vi "Create Arrow.vi"(6 "Quiver Size":sgl, 7 "Scale":cluster{"X":sgl, "Y":sgl, "Z":sgl}, 8 "error in (no error)":errorcluster, 9 "Color Array":cluster{"R":sgl, "G":sgl, "B":sgl, "A":sgl}[](array[cluster]), 10 "Normal Vertex":cluster{"X":sgl, "Y":sgl, "Z":sgl}[](array[cluster]), 11 "Quiver Object In":refnum<vi>) -> (0 "error out":errorcluster, 3 "Quiver Object Out":refnum<vi>)   [LabVIEW 2017, in "3D Quiver.lvclass"]
uses:
  <vilib>/Math Plots/3D Math Plots/3D Quiver/3D Quiver/3D Quiver.lvclass
  <vilib>/picture/3D Picture Control/Object/Create Object (name).vi
  <vilib>/picture/3D Picture Control/NI_3D Picture Control.lvlib
  <vilib>/Math Plots/3D Math Plots/3D Plot/3D Plot/3D Plot.lvclass
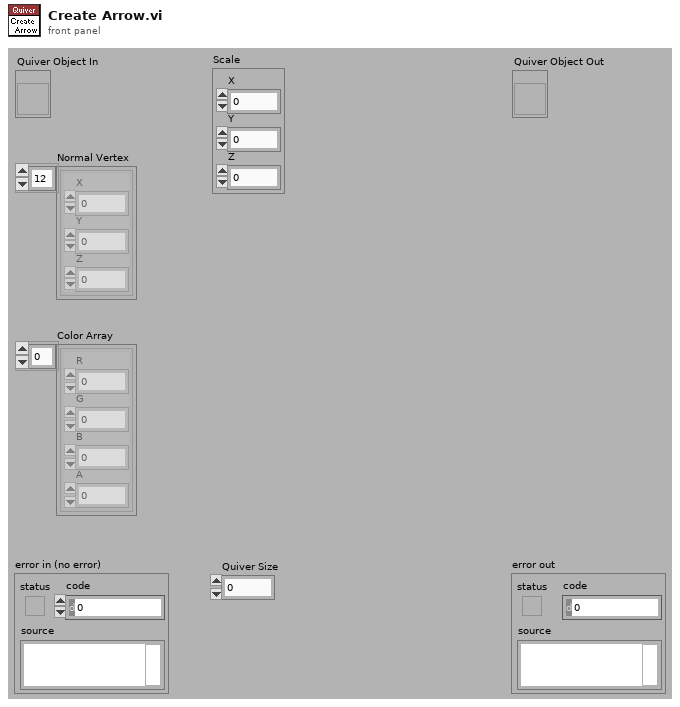
[diagram p1: front panel]
types:
  T1 = enum16{"Overall", "Per Primitive", "Per Vertex", "Binding Off"}
  T2 = enum16{"Points", "Lines", "Line Strip", "Line Loop", "Triangles", "Triangle Strip", "Triangle Fan", "Quads", "Quad Strip", "Polygon"}
  T3 = enum16{"Inherit Value", "Points", "Wireframe", "Polygons"}
  T4 = enum16{"Normal Bin", "Opaque Bin", "Transparent Bin"}
  T5 = cluster{"Product[0]":sgl, "Product[1]":sgl, "Product[2]":sgl}
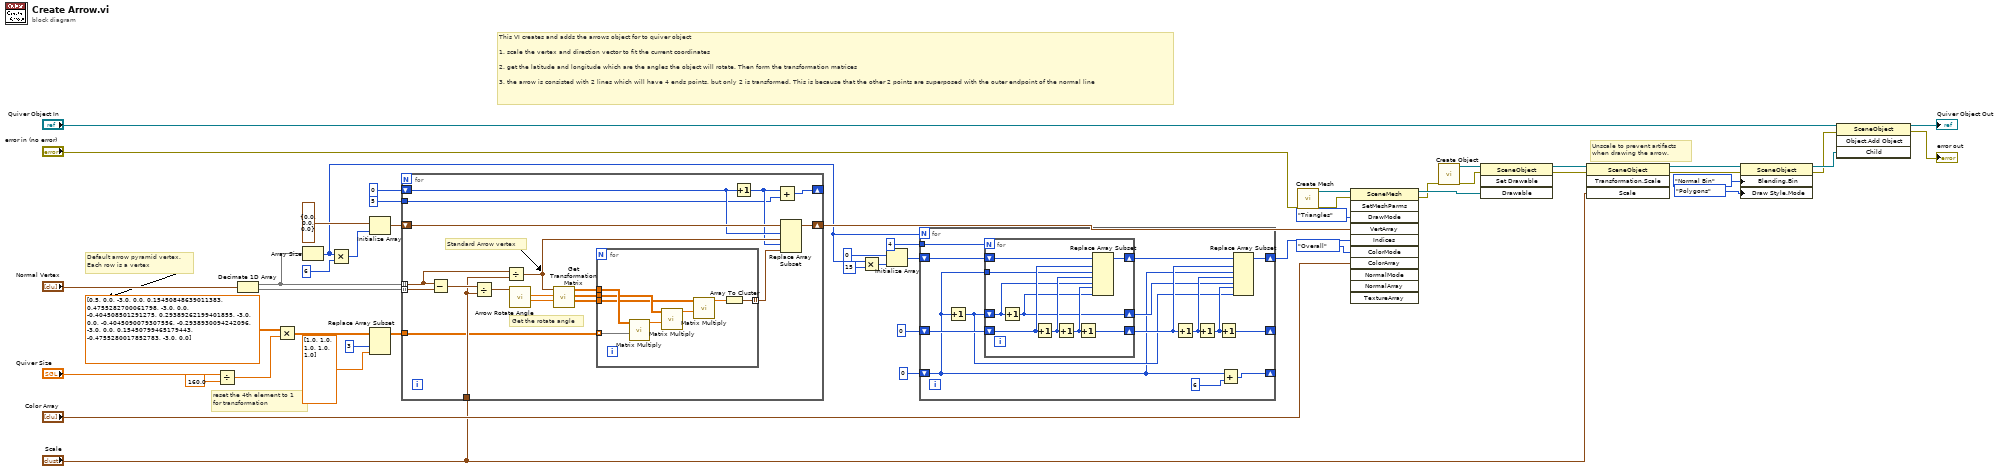
[diagram p0: block diagram]
diagram:
  # "reset the 4th element to 1 \nfor transformation"
  # "Default arrow pyramid vertex.\nEach row is a vertex"
  # "This VI creates and adds the arrows object for to quiver object\n\n1. scale the vertex and direction vector to fit the current coordinates\n\n2. get the latitude and longitude which are the angles the object will rotate. Then form the transformation matrices\n\n3. the arrow is consisted with 2 lines which will have 4 ends points, but only 2 is transformed. This is because that the other 2 points are superposed with the outer endpoint of the normal line"
  # "Unscale to prevent artifacts \nwhen drawing the arrow."
  n1 = Divide(x="Quiver Size", y=sgl 160.0) -> (x/y=w20:sgl)
  n2 = Decimate 1D Array("Normal Vertex") -> (w28:cluster{"X":sgl, "Y":sgl, "Z":sgl}[], w18:cluster{"X":sgl, "Y":sgl, "Z":sgl}[])
  n3 = Multiply(x=sgl[][] [[0.5, 0.0, -3.0, 0.0], [0.15450849, 0.47552827, -3.0, 0.0], [-0.4045085, 0.29389262, -3.0, 0.0], [-0.404509, -0.293893, -3.0, 0.0], [0.154508, -0.475528, -3.0, 0.0]], y=w20) -> (x*y=w24:sgl[][])
  n4 = Array Size(array=w28) -> (size(s)=w6:i32)
  n5 = Multiply(x=w6, y=6) -> (x*y=w31:i32)
  n6 = Initialize Array(cluster{"X":sgl, "Y":sgl, "Z":sgl} {"X"=0.0, "Y"=0.0, "Z"=0.0} ("Vector"), w31) -> (w29:cluster{"X":sgl, "Y":sgl, "Z":sgl}[])
  n7 = Replace Array Subset(array=w24, new element=sgl[] [1.0, 1.0, 1.0, 1.0, 1.0] ("new element/subarray"), index (col)=3 ("index (row)")) -> (w26:sgl[][])  [unwired: 1 in]
  n8 = for {
    tunnel: w28 -> [w60] mode=indexing
    tunnel: w18 -> [w67] mode=indexing
    tunnel: "Scale" -> [w59]
    shift-right: [w56] -> w21
    shift-left: w29 -> [w57]
    tunnel: w26 -> [w58]
    shift-right: [w51] -> _
    shift-left: 0 ("y") -> [w53]
    tunnel: 5 ("y") -> [w50]
    # "Standard Arrow vertex"
    # "Get the rotate angle"
    n9 = Subtract(x=w60, y=w67) -> (x-y=w68:cluster{"X":sgl, "Y":sgl, "Z":sgl})
    n10 = Divide(x=w68, y=w59) -> (x/y=w66:cluster{"X":sgl, "Y":sgl, "Z":sgl})
    n11 = Divide(x=w60, y=w59) -> (x/y=w54:cluster{"X":sgl, "Y":sgl, "Z":sgl})
    n12 = call <vilib>:"Arrow Rotate Angle.vi"("Vector"=w66) -> ("Z Axis Rotate Angle"=w64:sgl, "Y Axis Rotate Angle"=w65:sgl)  [unwired: 9 out]
    n13 = call <vilib>:"Get Transformation Matrix.vi"("Z Axis Rotate Angle"=w64, "Y Axis Rotate Angle"=w65, "Quiver Vector"=w54) -> ("Transtlate to Quiver Vertex"=w61:sgl[][], "Rotate by Z Axis"=w62:sgl[][], "Rotate by Y Axis"=w63:sgl[][])  [unwired: 6 out]
    n14 = for {
      tunnel: w63 -> [w76]
      tunnel: w62 -> [w75]
      tunnel: w61 -> [w72]
      tunnel: w58 -> [w69] mode=indexing
      tunnel: [w70] -> w55 mode=indexing
      n15 = call <vilib>:"Matrix Multiply.vi"("Vector"=w69, "Matrix"=w76) -> ("Product"=w74:sgl[])  [unwired: 9 out]
      n16 = call <vilib>:"Matrix Multiply.vi"("Vector"=w74, "Matrix"=w75) -> ("Product"=w73:sgl[])  [unwired: 9 out]
      n17 = call <vilib>:"Matrix Multiply.vi"("Vector"=w73, "Matrix"=w72) -> ("Product"=w71:sgl[])  [unwired: 9 out]
      n18 = Array To Cluster(array=w71) -> (cluster=w70:T5)
    }
    n19 = Increment(x=w53) -> (x+1=w52:i32)
    n20 = Add(x=w52, y=w50) -> (x+y=w51:i32)
    n21 = Replace Array Subset(array=w57, new element #1=w54, index #1=w53, new element #2=w55, index #2=w52) -> (w56:cluster{"X":sgl, "Y":sgl, "Z":sgl}[])
  }
  n22 = Multiply(x=w6, y=15) -> (x*y=w8:i32)
  n23 = Initialize Array(u32 0 ("unsigned 32bit integer"), w8) -> (w7:u32[])
  n24 = for {
    N: w6 -> [_]
    shift-right: [w87] -> w22
    shift-left: w7 -> [w90]
    shift-right: [w86] -> _
    shift-left: 0 -> [w89]
    shift-right: [w79] -> _
    shift-left: u32 0 -> [w78]
    tunnel: 4 -> [w77]
    n25 = Increment(x=w78) -> (x+1=w81:u32)
    n26 = for {
      N: w77 -> [_]
      shift-right: [w98] -> w88
      shift-left: w90 -> [w99]
      shift-right: [w94] -> w83
      shift-left: w89 -> [w95]
      tunnel: w78 -> [w93]
      shift-right: [w92] -> w82
      shift-left: w81 -> [w91]
      n27 = Increment(x=w91) -> (x+1=w92:u32)
      n28 = Increment(x=w95) -> (x+1=w96:i32)
      n29 = Increment(x=w96) -> (x+1=w97:i32)
      n30 = Increment(x=w97) -> (x+1=w94:i32)
      n31 = Replace Array Subset(array=w99, new element #1=w93, index #1=w95, new element #2=w91, index #2=w96, new element #3=w92, index #3=w97) -> (w98:u32[])
    }
    n32 = Increment(x=w83) -> (x+1=w84:i32)
    n33 = Increment(x=w84) -> (x+1=w85:i32)
    n34 = Increment(x=w85) -> (x+1=w86:i32)
    n35 = Add(x=w78, y=u32 6 ("x")) -> (x+y=w79:u32)
    n36 = Replace Array Subset(array=w88, new element #1=w78, index #1=w83, new element #2=w82, index #2=w84, new element #3=w81, index #3=w85) -> (w87:u32[])
  }
  n37 = call <vilib>:"Create Mesh.vi"("error in (no error)"="error in (no error)") -> ("error out"=w15:errorcluster, "New Mesh Refnum"=w14:refnum<vi>)  [unwired: 9 out]
  n38 = invoke class="SceneMesh" method="SetMeshParms"(reference=w14, error in=w15, "DrawMode"=T2."Triangles" ("Draw Mode"), "VertArray"=w21, "Indices"=w22, "ColorMode"=T1."Overall" ("Color Binding Mode"), "ColorArray"="Color Array") -> (reference out=w13:refnum<vi>, error out=w12:errorcluster)  [unwired: 4 in, 9 out]
  n39 = call-poly <vilib>:"Create Object.vi"("error in (no error)"=w12) -> ("error out"=w10:errorcluster, "Scene:New Object"=w11:refnum<vi>)  [unwired: 9 in]
  n40 = invoke class="SceneObject" method="Set Drawable"(reference=w11, error in=w10, "Drawable"=w13) -> (reference out=w35:refnum<vi>, error out=w34:errorcluster)  [unwired: 1 in, 2 out]
  n41 = invoke class="SceneObject" method="Transformation.Scale"(reference=w35, error in=w34, "Scale"="Scale") -> (reference out=w43:refnum<vi>, error out=w42:errorcluster)  [unwired: 1 in, 2 out]
  n42 = property class="SceneObject"(reference=w43, error in=w42, "Blending.Bin"=T4."Normal Bin" ("Blending:Bin"), "Draw Style.Mode"=T3."Polygons" ("Draw Style:Mode")) -> (reference out=w45:refnum<vi>, error out=w44:errorcluster)
  n43 = invoke class="SceneObject" method="Object.Add Object"(reference="Quiver Object In", error in=w44, "Child"=w45) -> (reference out=→"Quiver Object Out":refnum<vi>, error out=→"error out":errorcluster)  [unwired: 1 in, 2 out]
